vi "Timestamp.vi"   [LabVIEW 2019]
uses:
  <vilib>/rvi/Emulation/niFpgaGetClockAttributes.vi
  <vilib>/rvi/Emulation/niFpgaSctlEmulationGetInTimedLoop.vi
  <vilib>/rvi/Emulation/niFpgaEmulationReportErrorSimple.vi
  <vilib>/rvi/eio/common/nirviEmuTemplateMethod_errors.vi
  <vilib>/rvi/interface/RandomDataEmulation/niFpgaRandomDataHandleErrors.vi
  <vilib>/rvi/Emulation/niFpgaEmulationIsFPGAContextNoSignature.vi
  <vilib>/rvi/DataTransferAndStorage/Container/Common/niFpgaContainerGetUniqueNameForEmu.vi
  <vilib>/rvi/Memory/Memory_Emulation/niFpgaMemoryEmulationCacheClearOnFirstRun.vi
  <vilib>/rvi/Memory/Memory_Emulation/nirvimemoryEmulationManagerCache_MakeExclusive.vi
  <vilib>/rvi/Memory/Memory_Emulation/niFpgaMemoryEmulationValidateCache.vi
  <vilib>/rvi/Memory/Memory_Emulation/nirvimemoryEmulationManagerCache_InsertValue.vi
  <vilib>/Utility/error.llb/Clear Errors.vi
  <vilib>/rvi/Memory/Memory_Emulation/nirvimemoryEmulationManagerCache_ReleaseExclusive.vi
  <vilib>/rvi/Memory/Memory_Emulation/nirvimemoryEmulationManagerCache_GetValue.vi
  <vilib>/rvi/Memory/Memory_Emulation/nirvimemoryEmulationManagerCache_SetValue.vi
  <vilib>/rvi/Emulation/niFpgaProcessEmulError.vi
  <vilib>/rvi/Emulation/niFpgaCriticalErrorInLSC.vi
  <vilib>/eio/EIONode/EIONode.xnode
  <vilib>/rvi/DataTransferAndStorage/Container/XNode/niFpgaContainer.xnode
  <vilib>/rvi/interface/RandomDataEmulation/nirviRandomDataFpgaReadWriteTemplate.vi
  <vilib>/rvi/DataTransferAndStorage/Register/Emulation/niFpgaRegisterEmulation.vi
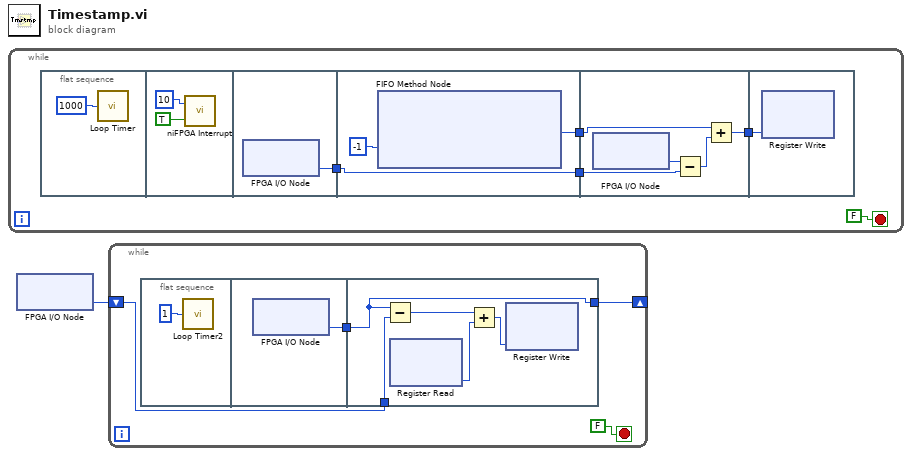
[diagram p0: block diagram]
diagram:
  n1 = while {
    stop <- FALSE stop-if-true
    n2 = flat-sequence {
      tunnel: [w10] -> w2
      tunnel: [w12] -> w6
      tunnel: w2 -> [w12]
      tunnel: [w11] -> w5
      tunnel: w6 -> [w17]
      tunnel: w5 -> [w15]
      tunnel: [w14] -> w4
      tunnel: w4 -> [w19]
      frame #0 {
        n3 = call "Loop Timer"("Count(mSec)"=u16 1000) -> ()  [unwired: 1 out]
      }
      frame #1 {
        n4 = call <vilib>:"niFPGA Interrupt.vi"("Wait Until Cleared (F)"=TRUE, "IRQ Number (0)"=u8 10) -> ()  [unwired: 1 in]
      }
      frame #2 {
        n5 = xnode "FPGA I/O Node"() -> ("Time"=w10:u64)  [unwired: 1 in, 1 out]
      }
      frame #3 {
        n6 = xnode ("FIFO Method Node")("Timeout"=-1) -> ("Element"=w11:u64)  [unwired: 1 in, 2 out]
      }
      frame #4 {
        n7 = xnode "FPGA I/O Node"() -> ("Time"=w18:u64)  [unwired: 1 in, 1 out]
        n8 = Subtract(x=w18, y=w17) -> (x-y=w16:u64)
        n9 = Add(x=w15, y=w16) -> (x+y=w14:u64)
      }
      frame #5 {
        n10 = xnode "Register Write"("Data"=w19) -> ()  [unwired: 1 in, 1 out]
      }
    }
  }
  n11 = xnode "FPGA I/O Node"() -> ("Time"=w1:u64)  [unwired: 1 in, 1 out]
  n12 = while {
    shift-right: [w23] -> _
    shift-left: w1 -> [w21]
    stop <- FALSE stop-if-true
    n13 = flat-sequence {
      tunnel: [w25] -> w22
      tunnel: [w27] -> w23
      tunnel: w22 -> [w27]
      tunnel: w21 -> [w26]
      frame #0 {
        n14 = call "Loop Timer2"("Count(uSec)"=u8 1 ("Count(mSec)")) -> ()  [unwired: 1 out]
      }
      frame #1 {
        n15 = xnode "FPGA I/O Node"() -> ("Time"=w25:u64)  [unwired: 1 in, 1 out]
      }
      frame #2 {
        n16 = Subtract(x=w27, y=w26) -> (x-y=w28:u64)
        n17 = xnode "Register Read"() -> ("Data"=w29:u64)  [unwired: 1 in, 1 out]
        n18 = Add(x=w28, y=w29) -> (x+y=w30:u64)
        n19 = xnode "Register Write"("Data"=w30) -> ()  [unwired: 1 in, 1 out]
      }
    }
  }
